vi "Convert cxd file.vi"(8 "error in (no error)":errorcluster, 11 "TomoConversion in":refnum<class "TomoConversion.lvclass">) -> (0 "error out":errorcluster, 3 "TomoConversion out":refnum<class "TomoConversion.lvclass">)   [LabVIEW 2012, in "TomoConversion.lvclass"]
uses:
  TomoConversion.lvclass
  TomoConversion.lvclass/TomoConversion.ctl
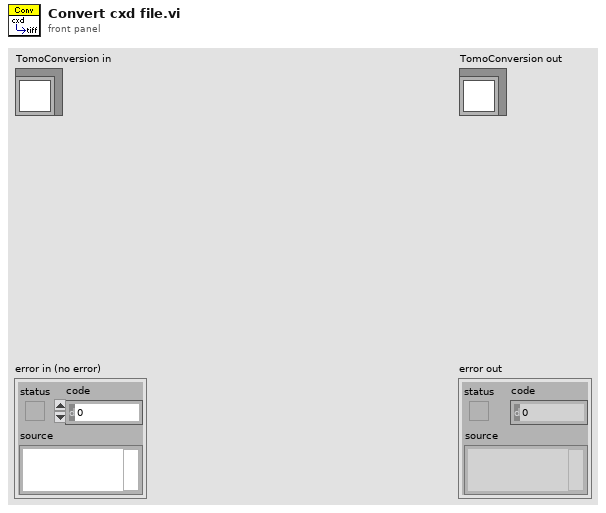
[diagram p1: front panel]
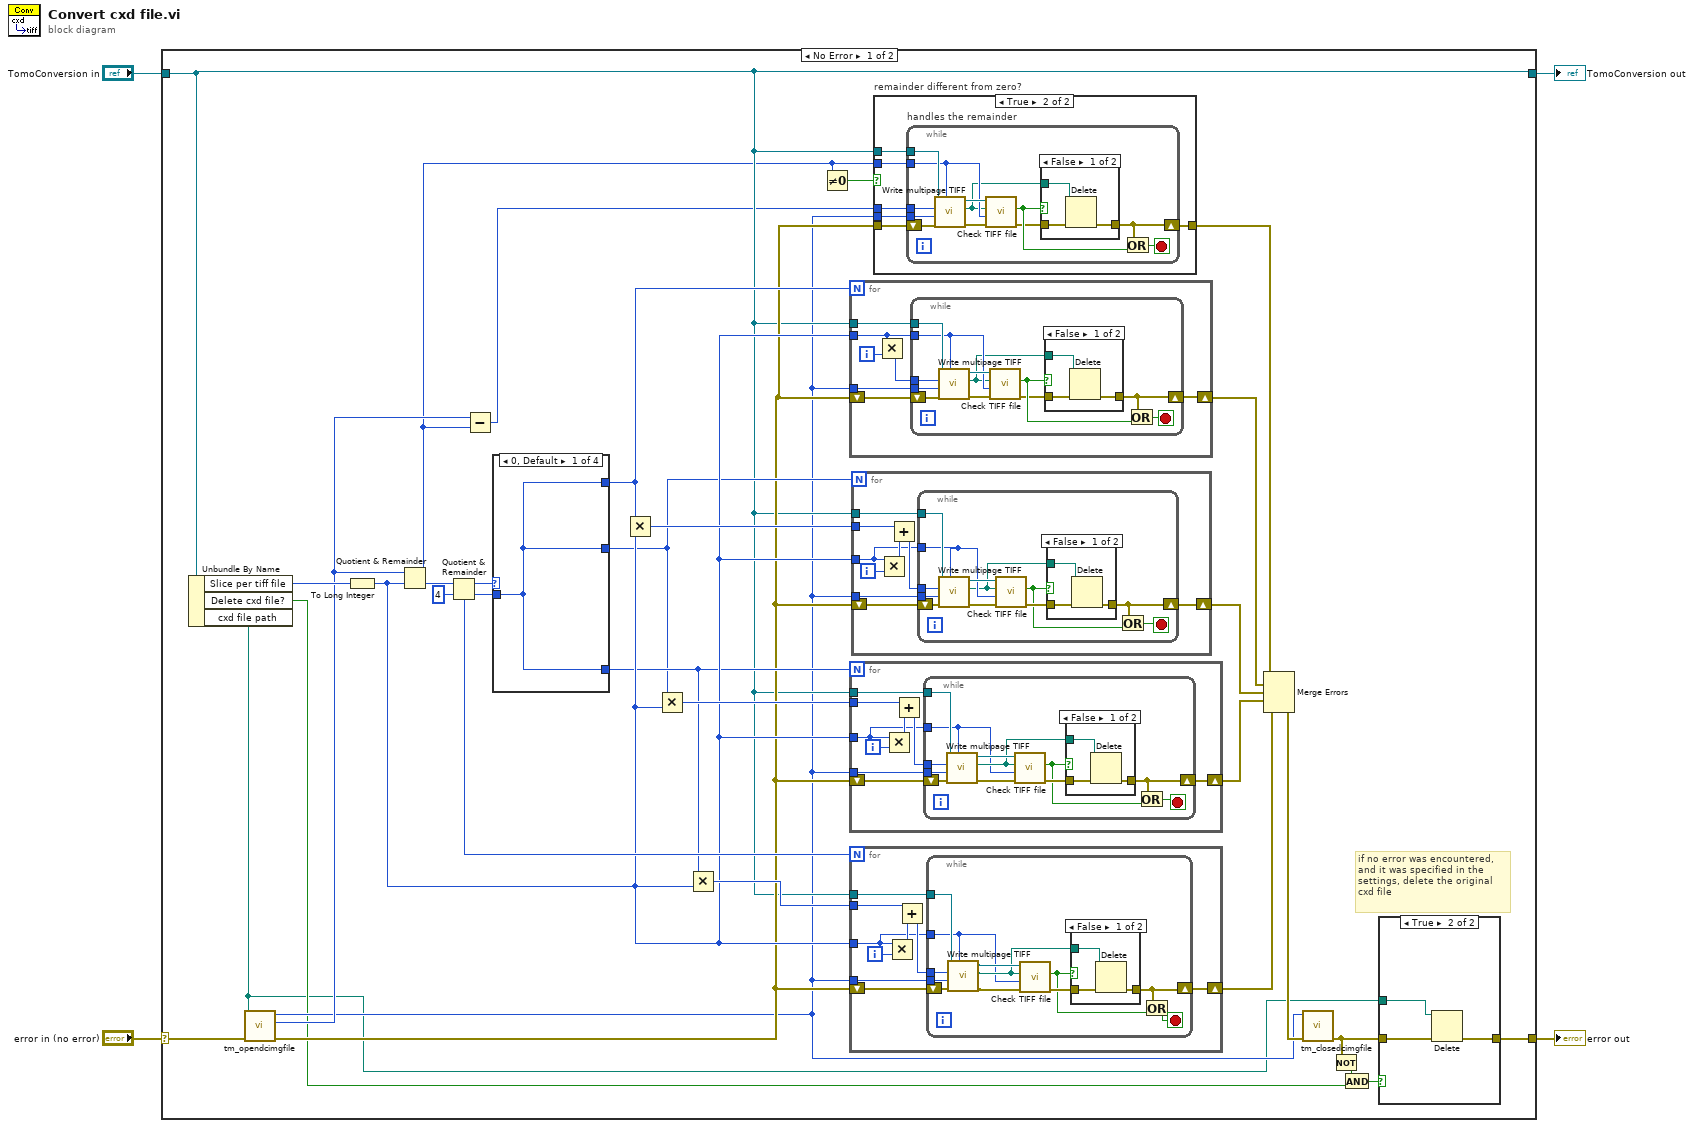
[diagram p0: block diagram]
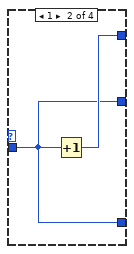
[diagram p5: hidden frame]
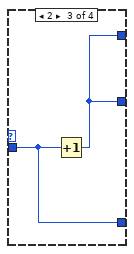
[diagram p6: hidden frame]
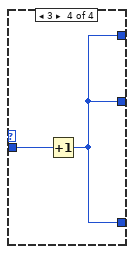
[diagram p7: hidden frame]
diagram:
  n1 = case shown="No Error" "error in (no error)" {
    selector: "error in (no error)" -> [w22 w170]
    tunnel: [w8 w170] -> w3
    tunnel: [w18 w169] -> w1
    tunnel: "TomoConversion in" -> [w18 w169]
    frame No Error {
      # "if no error was encountered, \nand it was specified in the \nsettings, delete the original\ncxd file"
      n2 = Unbundle By Name(w18) -> ("Slice per tiff file"=w36:u32, "Delete cxd file?"=w11:bool, "cxd file path"=w7:path)
      n3 = call <userlib>:"tm_opendcimgfile.vi"("error in (no error)"=w22, "Path"=w7) -> ("error out"=w19:errorcluster, "Total Frames"=w17:i32, "File Handle"=w13:u32)  [unwired: 7 in]
      n4 = To Long Integer(number=w36) -> (32bit integer=w27:i32)
      n5 = Quotient & Remainder(x=w17, y=w27) -> (x-y*floor(x/y)=w5:i32, floor(x/y)=w35:i32)
      n6 = Quotient & Remainder(x=w35, y=4) -> (x-y*floor(x/y)=w33:i32, floor(x/y)=w32:i32)
      n7 = Subtract(x=w17, y=w5) -> (x-y=w16:i32)
      n8 = case shown="0, Default" w33 {
        tunnel: w32 -> [w64 w65 w68 w70]
        tunnel: [w64 w66 w67 w69] -> w31
        tunnel: [w64 w65 w67 w69] -> w20
        tunnel: [w64 w65 w68 w69] -> w21
        frame 0, Default {
        }
        frame 1 {
          n9 = Increment(x=w65) -> (x+1=w66:i32)
        }
        frame 2 {
          n10 = Increment(x=w68) -> (x+1=w67:i32)
        }
        frame 3 {
          n11 = Increment(x=w70) -> (x+1=w69:i32)
        }
      }
      n12 = Multiply(x=w31, y=w27) -> (x*y=w30:i32)
      n13 = Multiply(x=w20, y=w27) -> (x*y=w29:i32)
      n14 = Multiply(x=w21, y=w27) -> (x*y=w28:i32)
      n15 = Not Equal To 0?(x=w5) -> (x != 0?=w6:bool)
      n16 = for {
        N: w31 -> [_]
        tunnel: w27 -> [w146]
        tunnel: w18 -> [w147]
        shift-right: [w151] -> w26
        shift-left: w19 -> [w150]
        tunnel: w13 -> [w149]
        i -> [w152]
        n17 = Multiply(x=w146, y=w152) -> (x*y=w148:i32)
        n18 = while {
          tunnel: w149 -> [w163]
          tunnel: w148 -> [w162]
          tunnel: w147 -> [w161]
          tunnel: w146 -> [w158]
          shift-right: [w153] -> w151
          shift-left: w150 -> [w164]
          stop <- w157 stop-if-true
          n19 = call-dynamic "Write multipage TIFF.vi"("number of TIFF slices"=w158, "error in (no error)"=w164, "cxd file handle"=w163, "offset"=w162, "TomoConversion in"=w161) -> ("error out"=w160:errorcluster, "TIFF file path"=w154:path, "TomoConversion out"=w159:refnum<class "TomoConversion.lvclass">)  [unwired: 4 in]
          n20 = call-dynamic "Check TIFF file.vi"("error in (no error)"=w160, "Expected TIFF slices"=w158, "TIFF File path"=w154, "TomoConversion in"=w159) -> ("error out"=w155:errorcluster, "is fine?"=w156:bool)  [unwired: 5 in, 1 out]
          n21 = case shown="False" w156 {
            tunnel: w155 -> [w167 w168]
            tunnel: w154 -> [w166 _]
            tunnel: [w165 w168] -> w153
            frame False {
              n22 = Delete(path (use dialog)=w166, error in=w167) -> (error out=w165:errorcluster)  [unwired: 3 in, 2 out]
            }
            frame True {
            }
          }
          n23 = Or(x=w153, y=w156) -> (x .or. y?=w157:bool)
        }
      }
      n24 = for {
        N: w21 -> [_]
        tunnel: w29 -> [w102]
        tunnel: w27 -> [w96]
        tunnel: w18 -> [w97]
        shift-right: [w100] -> w24
        shift-left: w19 -> [w101]
        tunnel: w13 -> [w99]
        i -> [w104]
        n25 = Multiply(x=w96, y=w104) -> (x*y=w103:i32)
        n26 = Add(x=w102, y=w103) -> (x+y=w98:i32)
        n27 = while {
          tunnel: w99 -> [w115]
          tunnel: w98 -> [w114]
          tunnel: w97 -> [w113]
          tunnel: w96 -> [w106]
          shift-right: [w109] -> w100
          shift-left: w101 -> [w116]
          stop <- w105 stop-if-true
          n28 = call-dynamic "Write multipage TIFF.vi"("number of TIFF slices"=w106, "error in (no error)"=w116, "cxd file handle"=w115, "offset"=w114, "TomoConversion in"=w113) -> ("error out"=w110:errorcluster, "TIFF file path"=w107:path, "TomoConversion out"=w108:refnum<class "TomoConversion.lvclass">)  [unwired: 4 in]
          n29 = call-dynamic "Check TIFF file.vi"("error in (no error)"=w110, "Expected TIFF slices"=w106, "TIFF File path"=w107, "TomoConversion in"=w108) -> ("error out"=w112:errorcluster, "is fine?"=w111:bool)  [unwired: 5 in, 1 out]
          n30 = case shown="False" w111 {
            tunnel: w112 -> [w119 w120]
            tunnel: w107 -> [w118 _]
            tunnel: [w117 w120] -> w109
            frame False {
              n31 = Delete(path (use dialog)=w118, error in=w119) -> (error out=w117:errorcluster)  [unwired: 3 in, 2 out]
            }
            frame True {
            }
          }
          n32 = Or(x=w109, y=w111) -> (x .or. y?=w105:bool)
        }
      }
      n33 = for {
        N: w32 -> [_]
        tunnel: w28 -> [w78]
        tunnel: w27 -> [w71]
        tunnel: w18 -> [w72]
        shift-right: [w75] -> w23
        shift-left: w19 -> [w76]
        tunnel: w13 -> [w74]
        i -> [w79]
        n34 = Multiply(x=w71, y=w79) -> (x*y=w77:i32)
        n35 = Add(x=w78, y=w77) -> (x+y=w73:i32)
        n36 = while {
          tunnel: w74 -> [w90]
          tunnel: w73 -> [w89]
          tunnel: w72 -> [w88]
          tunnel: w71 -> [w80]
          shift-right: [w84] -> w75
          shift-left: w76 -> [w91]
          stop <- w85 stop-if-true
          n37 = call-dynamic "Write multipage TIFF.vi"("number of TIFF slices"=w80, "error in (no error)"=w91, "cxd file handle"=w90, "offset"=w89, "TomoConversion in"=w88) -> ("error out"=w83:errorcluster, "TIFF file path"=w81:path, "TomoConversion out"=w82:refnum<class "TomoConversion.lvclass">)  [unwired: 4 in]
          n38 = call-dynamic "Check TIFF file.vi"("error in (no error)"=w83, "Expected TIFF slices"=w80, "TIFF File path"=w81, "TomoConversion in"=w82) -> ("error out"=w87:errorcluster, "is fine?"=w86:bool)  [unwired: 5 in, 1 out]
          n39 = case shown="False" w86 {
            tunnel: w87 -> [w94 w95]
            tunnel: w81 -> [w93 _]
            tunnel: [w92 w95] -> w84
            frame False {
              n40 = Delete(path (use dialog)=w93, error in=w94) -> (error out=w92:errorcluster)  [unwired: 3 in, 2 out]
            }
            frame True {
            }
          }
          n41 = Or(x=w84, y=w86) -> (x .or. y?=w85:bool)
        }
      }
      n42 = for {
        N: w20 -> [_]
        tunnel: w30 -> [w127]
        tunnel: w27 -> [w121]
        tunnel: w18 -> [w122]
        shift-right: [w126] -> w25
        shift-left: w19 -> [w125]
        tunnel: w13 -> [w124]
        i -> [w129]
        n43 = Multiply(x=w121, y=w129) -> (x*y=w128:i32)
        n44 = Add(x=w127, y=w128) -> (x+y=w123:i32)
        n45 = while {
          tunnel: w124 -> [w140]
          tunnel: w123 -> [w139]
          tunnel: w122 -> [w138]
          tunnel: w121 -> [w135]
          shift-right: [w131] -> w126
          shift-left: w125 -> [w141]
          stop <- w132 stop-if-true
          n46 = call-dynamic "Write multipage TIFF.vi"("number of TIFF slices"=w135, "error in (no error)"=w141, "cxd file handle"=w140, "offset"=w139, "TomoConversion in"=w138) -> ("error out"=w136:errorcluster, "TIFF file path"=w133:path, "TomoConversion out"=w137:refnum<class "TomoConversion.lvclass">)  [unwired: 4 in]
          n47 = call-dynamic "Check TIFF file.vi"("error in (no error)"=w136, "Expected TIFF slices"=w135, "TIFF File path"=w133, "TomoConversion in"=w137) -> ("error out"=w134:errorcluster, "is fine?"=w130:bool)  [unwired: 5 in, 1 out]
          n48 = case shown="False" w130 {
            tunnel: w134 -> [w144 w145]
            tunnel: w133 -> [w143 _]
            tunnel: [w142 w145] -> w131
            frame False {
              n49 = Delete(path (use dialog)=w143, error in=w144) -> (error out=w142:errorcluster)  [unwired: 3 in, 2 out]
            }
            frame True {
            }
          }
          n50 = Or(x=w131, y=w130) -> (x .or. y?=w132:bool)
        }
      }
      n51 = case "remainder different from zero?" shown="True" w6 {
        tunnel: w19 -> [w37 w43]
        tunnel: w18 -> [_ w42]
        tunnel: w5 -> [_ w41]
        tunnel: w16 -> [_ w40]
        tunnel: [w37 w39] -> w15
        tunnel: w13 -> [_ w38]
        frame False {
        }
        frame True {
          n52 = while "handles the remainder" {
            tunnel: w38 -> [w54]
            tunnel: w42 -> [w53]
            tunnel: w41 -> [w50]
            shift-right: [w45] -> w39
            shift-left: w43 -> [w55]
            tunnel: w40 -> [w44]
            stop <- w49 stop-if-true
            n53 = call-dynamic "Write multipage TIFF.vi"("number of TIFF slices"=w50, "error in (no error)"=w55, "cxd file handle"=w54, "offset"=w44, "TomoConversion in"=w53) -> ("error out"=w52:errorcluster, "TIFF file path"=w46:path, "TomoConversion out"=w51:refnum<class "TomoConversion.lvclass">)  [unwired: 4 in]
            n54 = call-dynamic "Check TIFF file.vi"("error in (no error)"=w52, "Expected TIFF slices"=w50, "TIFF File path"=w46, "TomoConversion in"=w51) -> ("error out"=w47:errorcluster, "is fine?"=w48:bool)  [unwired: 5 in, 1 out]
            n55 = case shown="False" w48 {
              tunnel: w47 -> [w58 w59]
              tunnel: w46 -> [w57 _]
              tunnel: [w56 w59] -> w45
              frame False {
                n56 = Delete(path (use dialog)=w57, error in=w58) -> (error out=w56:errorcluster)  [unwired: 3 in, 2 out]
              }
              frame True {
              }
            }
            n57 = Or(x=w45, y=w48) -> (x .or. y?=w49:bool)
          }
        }
      }
      n58 = Merge Errors(w15, w26, w25, w24, w23) -> (w14:errorcluster)
      n59 = call <userlib>:"tm_closedcimgfile.vi"("error in (no error)"=w14, "File Handle"=w13) -> ("error out"=w9:errorcluster)  [unwired: 9 in]
      n60 = Not(x=w9) -> (.not. x?=w12:bool)
      n61 = And(x=w12, y=w11) -> (x .and. y?=w10:bool)
      n62 = case shown="True" w10 {
        tunnel: w9 -> [w60 w63]
        tunnel: [w60 w62] -> w8
        tunnel: w7 -> [_ w61]
        frame False {
        }
        frame True {
          n63 = Delete(path (use dialog)=w61, error in=w63) -> (error out=w62:errorcluster)  [unwired: 3 in, 2 out]
        }
      }
    }
    frame Error {
    }
  }
  "error out" <- w3
  "TomoConversion out" <- w1
